vi "DBinfo.vi"(0 "Message":string, 1 "panelName":string) -> ()   [LabVIEW 2015]
uses:
  GlobalPath.vi
panel:
  out "DBpath":path=path "/home/atlas/Micromegas/M0Data/dbtxtfiles"
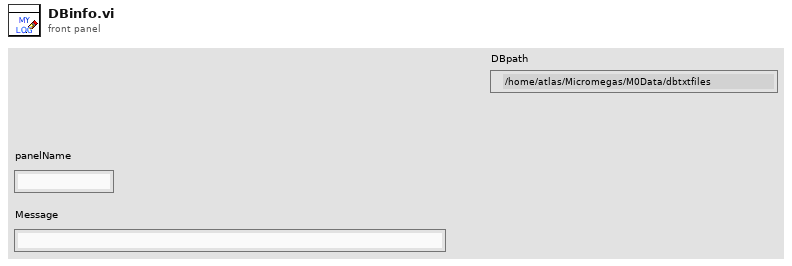
[diagram p1: front panel]
types:
  T1 = enum16{"open", "replace", "create", "open or create", "replace or create", "replace or create with confirmation"}
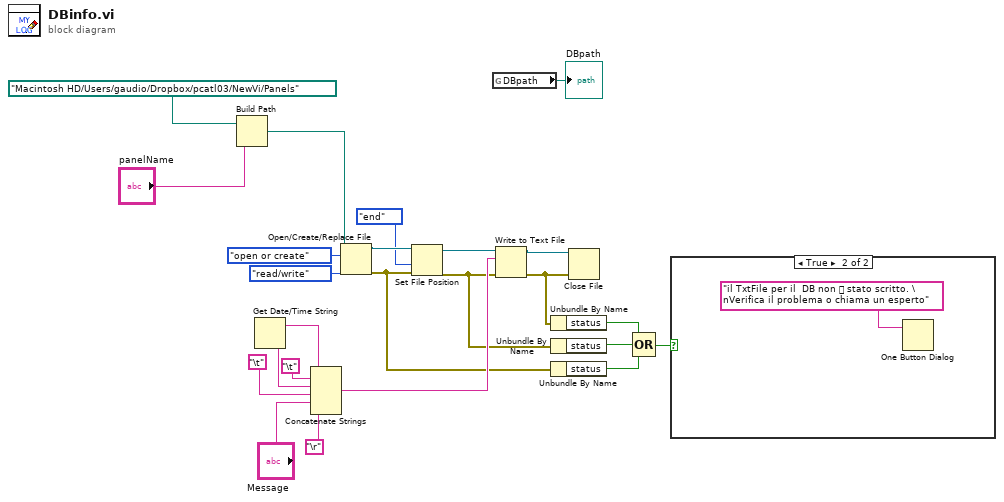
[diagram p0: block diagram]
diagram:
  n1 = Build Path(base path=path "/Macintosh HD/Users/gaudio/Dropbox/pcatl03/NewVi/Panels" ("path"), name or relative path="panelName") -> (appended path=w13:path)
  n2 = Get Date/Time String() -> (date string=w17:string, time string=w16:string)  [unwired: 3 in]
  n3 = Concatenate Strings(w17, "\t", w16, "\t", "Message", "\r") -> (w19:string)
  n4 = Open/Create/Replace File(file path (use dialog)=w13, operation (0:open)=T1."open or create", access (0:read/write)=enum16{"read/write", "read-only", "write-only"}."read/write") -> (refnum out=w21:refnum<file>, error out=w8:errorcluster)  [unwired: 3 in, 1 out]
  n5 = Set File Position(refnum=w21, from (0:start)=enum16{"start", "end", "current"}."end", error in=w8) -> (refnum out=w20:refnum<file>, error out=w7:errorcluster)  [unwired: 1 in]
  n6 = global read "GlobalPath.vi" "DBpath"() -> (→"DBpath":path)
  n7 = Write to Text File(file (use dialog)=w20, text=w19, error in=w7) -> (refnum out=w23:refnum<file>, error out=w9:errorcluster)  [unwired: 1 in, 1 out]
  n8 = Unbundle By Name(w9) -> ("status"=w6:bool)
  n9 = Unbundle By Name(w7) -> ("status"=w5:bool)
  n10 = Unbundle By Name(w8) -> ("status"=w4:bool)
  n11 = Close File(refnum=w23, error in=w9) -> ()  [unwired: 2 out]
  n12 = Compound Arithmetic op=OR(w6, w5, w4) -> (w3:bool)
  n13 = case shown="True" w3 {
    frame False {
    }
    frame True {
      n14 = One Button Dialog(message="il TxtFile per il  DB non  stato scritto. \nVerifica il problema o chiama un esperto") -> ()  [unwired: 1 in, 1 out]
    }
  }
